vi "RandomInt.vi"(10 "Min":i32, 11 "Max":i32) -> (3 "Random":i32)   [LabVIEW 2013]
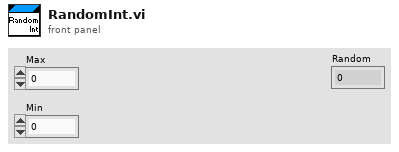
[diagram p1: front panel]
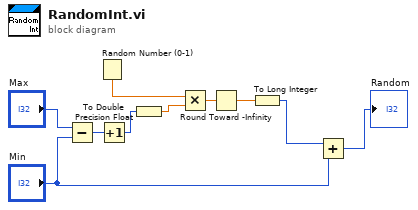
[diagram p0: block diagram]
diagram:
  n1 = Subtract(x="Max", y="Min") -> (x-y=w6:i32)
  n2 = Random Number (0-1)() -> (number: 0 to 1=w8:dbl)
  n3 = Increment(x=w6) -> (x+1=w5:i32)
  n4 = To Double Precision Float(number=w5) -> (double precision float=w4:dbl)
  n5 = Multiply(x=w8, y=w4) -> (x*y=w3:dbl)
  n6 = Round Toward -Infinity(1:w3) -> (0:w2:dbl)
  n7 = To Long Integer(number=w2) -> (32bit integer=w1:i32)
  n8 = Add(x=w1, y="Min") -> (x+y=→"Random":i32)
